vi "Read Motor Position.vi"(8 "error in (no error)":errorcluster, 10 "Motor ID (0)":u8, 11 "Dynamixel Motor Simulator in":refnum<class "Dynamixel Motor Simulator.lvclass">) -> (0 "error out":errorcluster, 2 "Position (deg)":dbl, 3 "Dynamixel Motor Simulator out":refnum<class "Dynamixel Motor Simulator.lvclass">)   [LabVIEW 2016, in "Dynamixel Motor Simulator.lvclass"]
doc: "Reads the motor's position."
uses:
  <instrlib>/Dynamixel Motor/HAIOL/Simulator/Dynamixel Motor Simulator.lvclass
  <instrlib>/Dynamixel Motor/HAIOL/Simulator/Dynamixel Motor Simulator.lvclass/Dynamixel Motor Simulator.ctl
  <vilib>/robotics/Simulator/Robot Factory/Motor/ODESimulator_Motor.lvclass
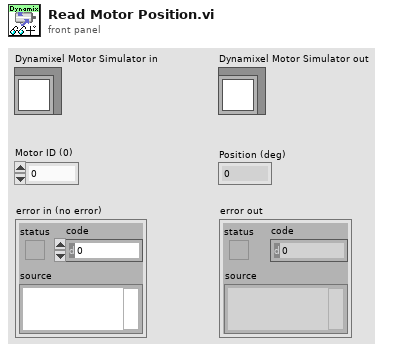
[diagram p1: front panel]
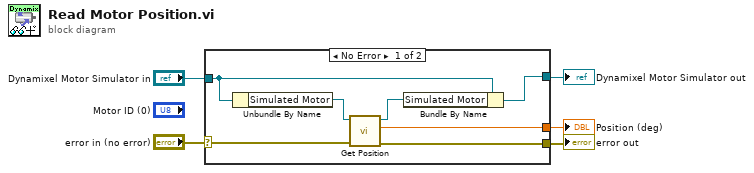
[diagram p0: block diagram]
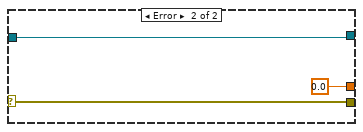
[diagram p2: hidden frame]
diagram:
  n1 = case shown="No Error" "error in (no error)" {
    selector: "error in (no error)" -> [w10 w14]
    tunnel: "Dynamixel Motor Simulator in" -> [w12 w15]
    tunnel: [w11 w15] -> w3
    tunnel: [w9 w14] -> w2
    tunnel: [w6 0.0 ("CCW Position (rad)")] -> w1
    frame No Error {
      n2 = Unbundle By Name(w12) -> ("Simulated Motor"=w7:refnum<class "ODESimulator_Motor.lvclass">)
      n3 = call-dynamic "Get Position.vi"("error in (no error)"=w10, "Motor in"=w7) -> ("error out"=w9:errorcluster, "CCW Position (rad)"=w6:dbl, "Motor out"=w8:refnum<class "ODESimulator_Motor.lvclass">)  [unwired: 7 in]
      n4 = Bundle By Name(cluster=w12, "Simulated Motor"=w8) -> (w11:refnum<class "Dynamixel Motor Simulator.lvclass">)
    }
    frame Error {
    }
  }
  "error out" <- w2
  "Dynamixel Motor Simulator out" <- w3
  "Position (deg)" <- w1
